vi "DAQtest.vi"() -> ()   [LabVIEW 2020]
uses:
  <vilib>/DAQmx/write.llb/DAQmx Write.vi
  <vilib>/DAQmx/write.llb/DAQmx Write (Analog 1D Wfm NChan NSamp).vi
  <vilib>/DAQmx/create/channels.llb/DAQmx Create Channel (AO-Voltage-Basic).vi
  <vilib>/DAQmx/configure/timing.llb/DAQmx Timing (Sample Clock).vi
  <vilib>/DAQmx/miscellaneous.llb/DAQmx Fill In Error Info.vi
  <resource>/objmgr/daqmx.rc
panel:
  in  "error in":errorcluster
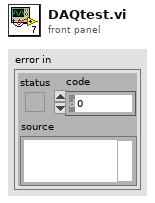
[diagram p1: front panel]
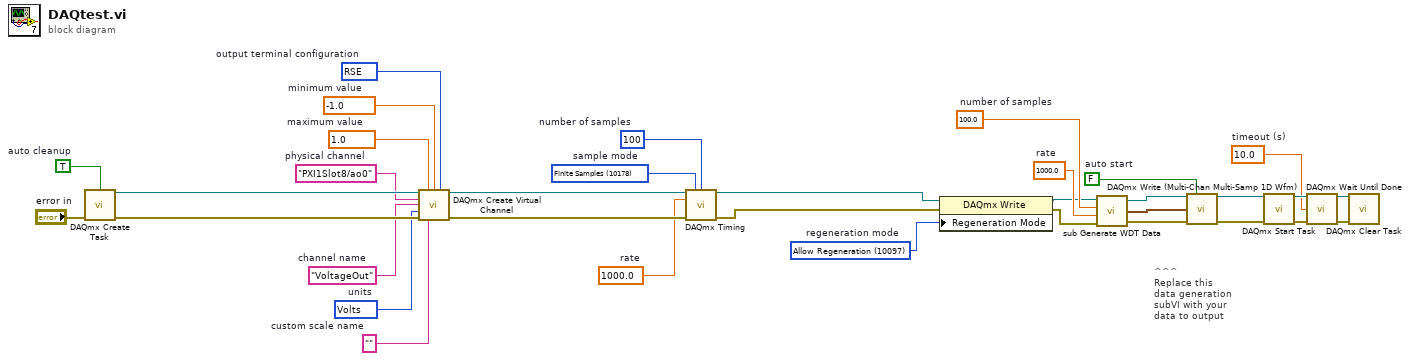
[diagram p0: block diagram]
diagram:
  w3 = 10097 items=["Allow Regeneration"=10097, "Do Not Allow Regeneration"=10158]  # regeneration mode
  w5 = 10178 items=["Finite Samples"=10178, "Continuous Samples"=10123, "Hardware Timed Single Point"=12522]  # sample mode
  w6 = 100  # number of samples
  w7 = 1000.0  # rate
  w10 = 10083 items=["Default"=-1, "RSE"=10083, "Differential"=10106, "Pseudodifferential"=12529]  # output terminal configuration
  w11 = 10348 items=["Volts"=10348, "From Custom Scale"=10065]  # units
  w12 = "VoltageOut"  # channel name
  w14 = ""  # custom scale name
  w15 = -1.0  # minimum value
  w16 = 1.0  # maximum value
  w17 = "PXI1Slot8/ao0"  # physical channel
  w19 = TRUE  # auto cleanup
  w25 = 10.0  # timeout (s)
  w29 = 1000.0  # rate
  w30 = 100.0  # number of samples
  w34 = FALSE  # auto start
  # "^^^\nReplace this\ndata generation\nsubVI with your\ndata to output"
  n1 = call <vilib>:"DAQmx Create Task.vi"("auto cleanup"=w19, "error in"="error in") -> ("task out"=w18:refnum<k21>, "error out"=w20:errorcluster)  [unwired: 12 in]
  n2 = call-poly <vilib>:"DAQmx Create Virtual Channel.vi"("task in"=w18, "maximum value"=w16, "minimum value"=w15, "output terminal configuration"=w10, "physical channels"=w17, "name to assign"=w12, "units"=w11, "error in"=w20, "custom scale name"=w14) -> ("task out"=w8:refnum<k21>, "error out"=w13:errorcluster)  [unwired: 5 in]
  n3 = call-poly <vilib>:"DAQmx Timing.vi"("task/channels in"=w8, "sample mode"=w5, "samples per channel"=w6, "rate"=w7, "error in"=w13) -> ("task out"=w4:refnum<k21>, "error out"=w9:errorcluster)  [unwired: 9 in]
  n4 = property class="DAQmx Write"(reference=w4, error in=w9, "Regeneration Mode"=w3) -> (reference out=w1:refnum<k21>, error out=w2:errorcluster)
  n5 = call <vilib>:"sub Generate WDT Data.vi"("task in"=w1, "number of samples"=w30, "update rate"=w29, "error in"=w2) -> ("task out"=w32:refnum<k21>, "Data"=w31:waveform(dbl)[], "error out"=w33:errorcluster)  [unwired: 1 in]
  n6 = call-poly "DAQmx Write (Multi-Chan Multi-Samp 1D Wfm).vi"("task/channels in"=w32, "auto start"=w34, "data"=w31, "error in"=w33) -> ("task out"=w24:refnum<k21>, "error out"=w23:errorcluster)  [unwired: 9 in, 1 out]
  n7 = call <vilib>:"DAQmx Start Task.vi"("task/channels in"=w24, "error in"=w23) -> ("task out"=w28:refnum<k21>, "error out"=w27:errorcluster)  [unwired: 12 in]
  n8 = call <vilib>:"DAQmx Wait Until Done.vi"("task/channels in"=w28, "timeout (sec)"=w25, "error in"=w27) -> ("task out"=w22:refnum<k21>, "error out"=w26:errorcluster)  [unwired: 11 in]
  n9 = call <vilib>:"DAQmx Clear Task.vi"("task in"=w22, "error in"=w26) -> ()  [unwired: 13 in, 1 out]
